vi "Add Tx Generic Status Section.vi"(8 "error in":errorcluster, 11 "Section Ref in":T1 format="%.0x") -> (0 "error out":errorcluster, 1 "Tx Queue Status channel Refs":T1[](array[typedef]) format="%.0x", 2 "Tx Queue Status Section Ref out":T1 format="%.0x", 3 "Section Ref out":T1 format="%.0x")   [LabVIEW 2020, in "AIM ARINC 664 Scripting.lvlib"]
uses:
  AIM ARINC 664 Scripting.lvlib
  <vilib>/NI VeriStand/Custom Device API/Custom Device Item Ref.ctl
  Controls/Tx Generic Queue Status Enum.ctl
  Constants.vi
  <vilib>/Utility/Data Type/NI_Data Type.lvlib
  GUID Utility/AIM ARINC 664 GUID Utility.lvlib
  <vilib>/NI VeriStand/Custom Device API/Custom Device API.lvlib
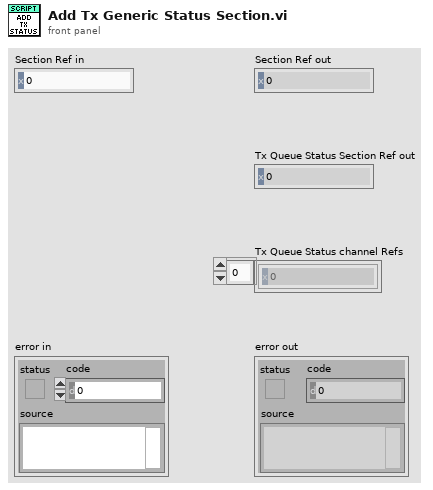
[diagram p1: front panel]
types:
  T1 = typedef "Custom Device API.lvlib/Custom Device Item Ref.ctl" = u64
  T2 = typedef "Tx Generic Queue Status Enum.ctl" = enum16{"FDX_QUE_EMPTY", "FDX_QUE_FILLED", "FDX_QUE_FULL", "FDX_QUE_SENT", "FDX_QUE_CYCL_RUN", "FDX_QUE_CYCL_SENT"}
  T3 = cluster{"Tx QueueStatus Channel":string, "enum names":string[], "Values":dbl[]}
  T4 = cluster{"Tx QueueStatus Channel":string, "enum names":string[], "Values":dbl[]}[]
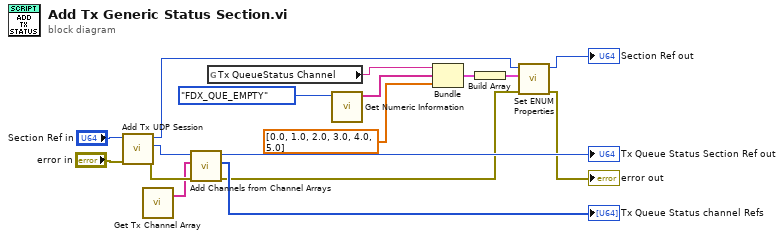
[diagram p0: block diagram]
diagram:
  n1 = call "Add Tx UDP Session.vi"("error in (no error)"="error in", "Section Ref in"="Section Ref in") -> ("error out"=w15:errorcluster, "Section Ptr"=w1:T1, "Parent Ref out"=w3:T1)  [unwired: 7 in]
  n2 = call "Get Tx Channel Array.vi"() -> ("Channel Array"=w7:string[])  [unwired: 3 in]
  n3 = call "Add Channels from Channel Arrays.vi"("error in"=w15, "Channel Array"=w7, "Section Ptr in"=w1) -> ("error out"=w5:errorcluster, "Channel Refs"=→"Tx Queue Status channel Refs":T1[], "Section Ptr out"=→"Tx Queue Status Section Ref out":T1)  [unwired: 6 in]
  n4 = global read "Constants.vi" "Tx QueueStatus Channel"() -> (w12:string)
  n5 = call <vilib>:"Get Numeric Information.vi"("variant"=Tx_Generic_Queue_Status_Enum."FDX_QUE_EMPTY") -> ("enum names"=w11:string[])  [unwired: 7 in, 3 out]
  n6 = Bundle("Tx QueueStatus Channel"=w12, "enum names"=w11, "Values"=dbl[] [0.0, 1.0, 2.0, 3.0, 4.0, 5.0]) -> (w9:T3)  [unwired: 1 in]
  n7 = Build Array(w9) -> (w13:T4)
  n8 = call "Set ENUM Properties.vi"("error in (no error)"=w5, "enum to be changes"=w13, "Parent Ref in"=w3) -> ("error out"=→"error out":errorcluster, "Parent Ref out"=→"Section Ref out":T1)  [unwired: 7 in]
